vi "USER_BarCode_Popup.vi"(0 "Enable":bool=TRUE, 5 "error in (no error)":errorcluster) -> (14 "UserBCPopup_ref_out":refnum<vi>, 17 "Bar Code":string, 18 "OK":bool, 19 "error out":errorcluster)   [LabVIEW 2018]
doc: "Displays a standard dialog box that prompts users to enter information, such as a user name and password.\n--------------------\n\nThis Express VI is configured as follows:\n\nMessage to Display to the User:Scan the WAM Barcode,\nThe bar code is located on the top of the WAM module\nThe inputs are: \nText Entry Box: Bar Code"
panel:
  in  "Bar Code":string
  out "String":string="Scan the Barcode on Your Employee Badge \nto Begin a New Session"
  in  "Cancel":bool
  in  "OK2":bool
  in  "OK1":bool
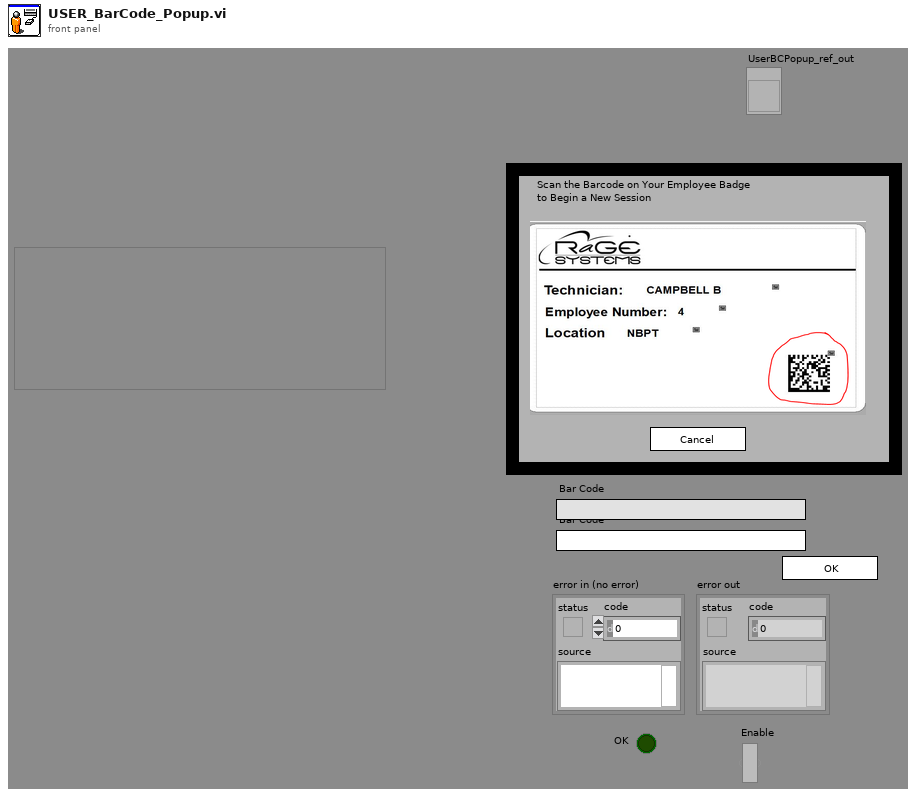
[diagram p1: front panel]
types:
  T1 = cluster{"Input Name":string, "Input Data Type":i32}[]
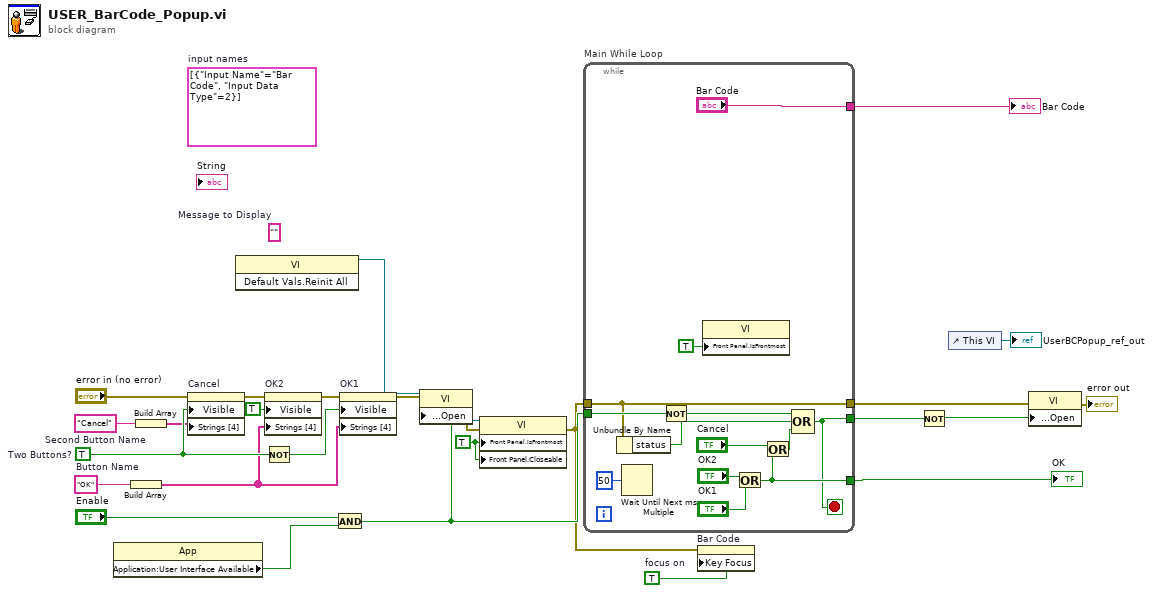
[diagram p0: block diagram]
diagram:
  w3 = TRUE ("Front Panel Window:Is Frontmost")
  w8 = TRUE  # focus on
  (unwired) T1 [{"Input Name"="Bar Code", "Input Data Type"=2}]  # input names
  w20 = "Cancel"  # Second Button Name
  w18 = "OK"  # Button Name
  (unwired) ""  # Message to Display
  w27 = TRUE  # Two Buttons?
  n1 = property class="App"() -> ("Application:User Interface Available"=w11:bool)  [unwired: 2 in, 2 out]
  n2 = Build Array(w18) -> (w19:string[])
  n3 = Build Array(w20) -> (w21:string[])
  n4 = property on="Cancel" class="Bool"(error in="error in (no error)", "Visible"=w27, "Strings [4]"=w21) -> (error out=w24:errorcluster)  [unwired: 1 in, 1 out]
  n5 = invoke class="VI" method="Default Vals.Reinit All"() -> (reference out=w10:refnum<vi>)  [unwired: 3 in, 2 out]
  n6 = Not(x=w27) -> (.not. x?=w25:bool)
  n7 = property on="OK2" class="Bool"(error in=w24, "Visible"=TRUE, "Strings [4]"=w19) -> (error out=w23:errorcluster)  [unwired: 1 in, 1 out]
  n8 = And(x="Enable", y=w11) -> (x .and. y?=w12:bool)
  n9 = property on="OK1" class="Bool"(error in=w23, "Visible"=w25, "Strings [4]"=w19) -> (error out=w17:errorcluster)  [unwired: 1 in, 1 out]
  n10 = property class="VI"(reference=w10, error in=w17, "Front Panel Window:Open"=w12) -> (reference out=w6:refnum<vi>, error out=w5:errorcluster)
  n11 = property class="VI"(reference=w6, error in=w5, "Front Panel.IsFrontmost"=w3, "Front Panel.Closeable"=w3) -> (error out=w4:errorcluster)  [unwired: 1 out]
  n12 = while "Main While Loop" {
    tunnel: [w37] -> w26
    tunnel: w12 -> [w35]
    tunnel: [w33] -> w22
    tunnel: w4 -> [w32]
    tunnel: [w32] -> w15
    tunnel: ["Bar Code"] -> w9
    stop <- w33 stop-if-true
    n13 = Unbundle By Name(w32) -> ("status"=w30:bool)
    n14 = Wait Until Next ms Multiple(millisecond multiple=u32 50) -> ()  [unwired: 1 out]
    n15 = Not(x=w35) -> (.not. x?=w34:bool)
    n16 = property class="VI"("Front Panel.IsFrontmost"=TRUE ("Front Panel Window:Is Frontmost")) -> ()  [unwired: 2 in, 2 out]
    n17 = Or(x="OK2", y="OK1") -> (x .or. y?=w37:bool)
    n18 = Or(x="Cancel", y=w37) -> (x .or. y?=w31:bool)
    n19 = Compound Arithmetic op=OR(w34, w30, w31) -> (w33:bool)
  }
  "OK" <- w26
  "Bar Code" <- w9
  n20 = property on="Bar Code" class="Str"(error in=w4, "Key Focus"=w8) -> ()  [unwired: 1 in, 2 out]
  n21 = Not(x=w22) -> (.not. x?=w7:bool)
  n22 = control-ref of="This VI"() -> (→"UserBCPopup_ref_out":refnum<vi>)
  n23 = property class="VI"(error in=w15, "Front Panel Window:Open"=w7) -> (error out=→"error out":errorcluster)  [unwired: 1 in, 1 out]
